vi "p32 zoom algoritmo.vi"() -> ()   [LabVIEW 2013]
panel:
  out "new picture 5":picture
  out "new picture 4":picture
  in  "Numeric 2":dbl
  out "new picture 3":picture
  in  "Numeric":dbl
  out "new picture 2":picture
  in  "path to BMP file":path
  out "new picture":picture
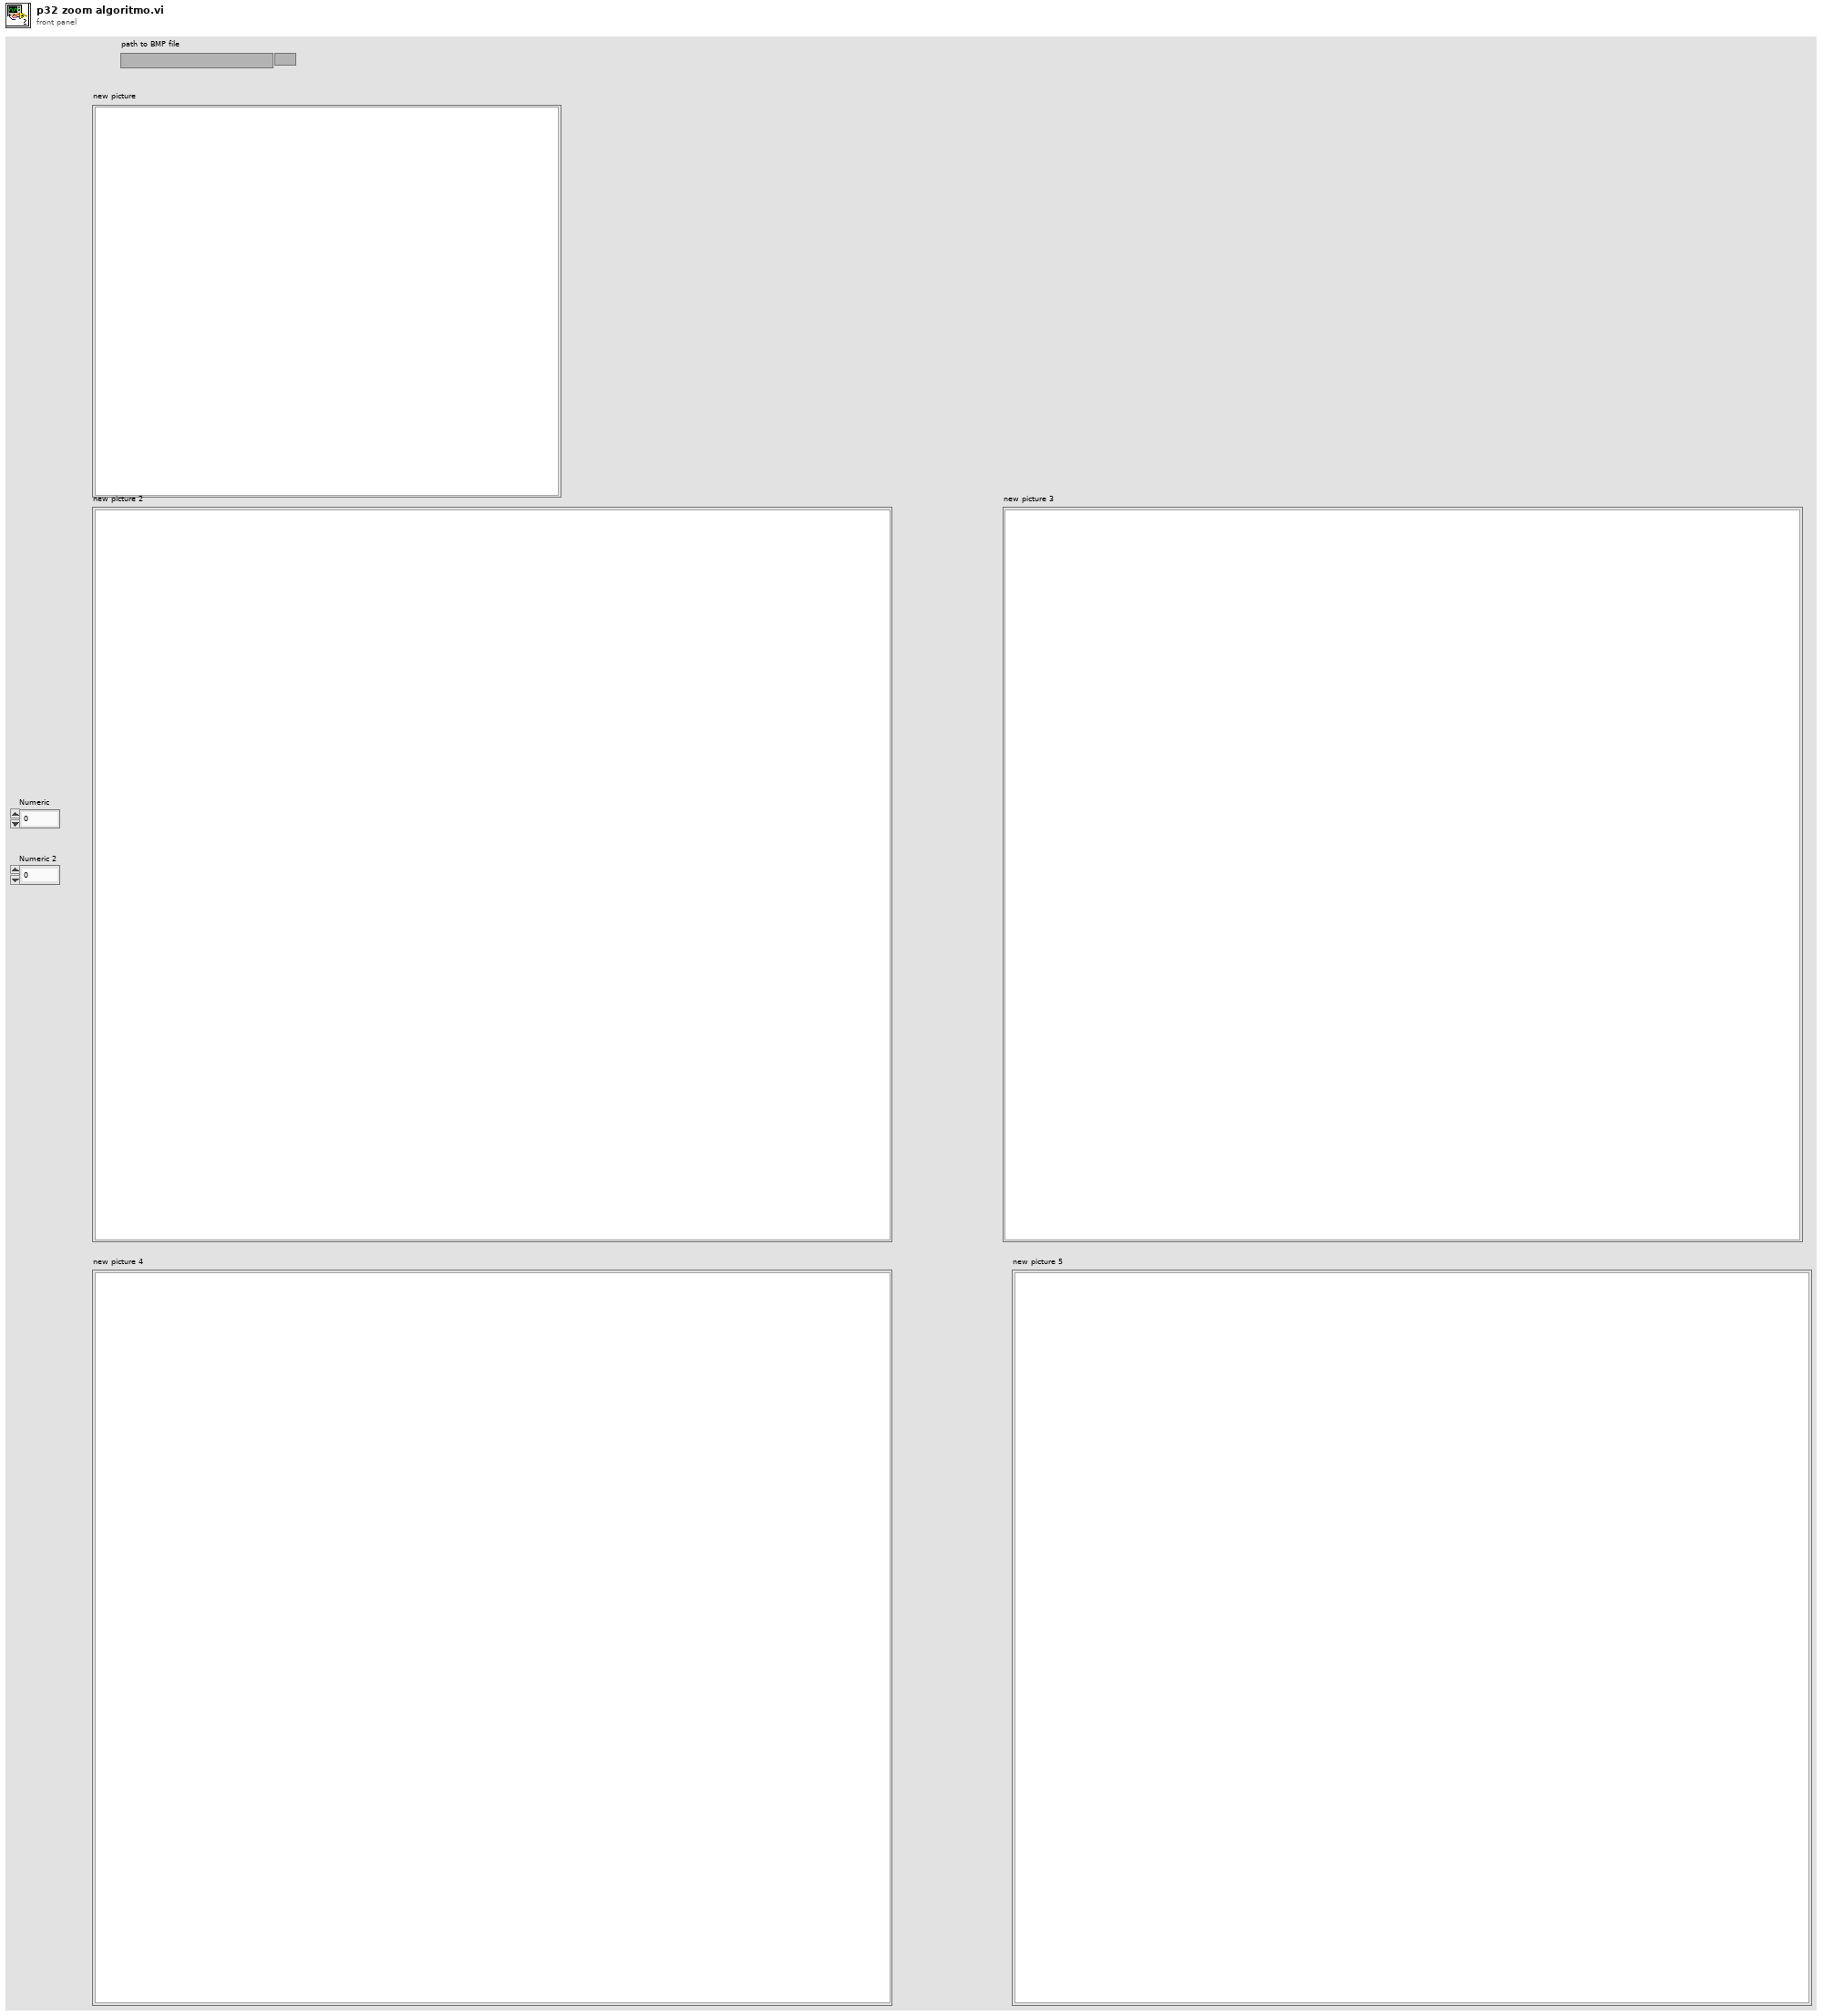
[diagram p1: front panel]
types:
  T1 = typedef "imagedata.ctl" = cluster{"image type":i32, "image depth":i32, "image":u8[], "mask":u8[], "colors":u32[], "Rectangle":cluster{"left":i16, "top":i16, "right":i16, "bottom":i16}}
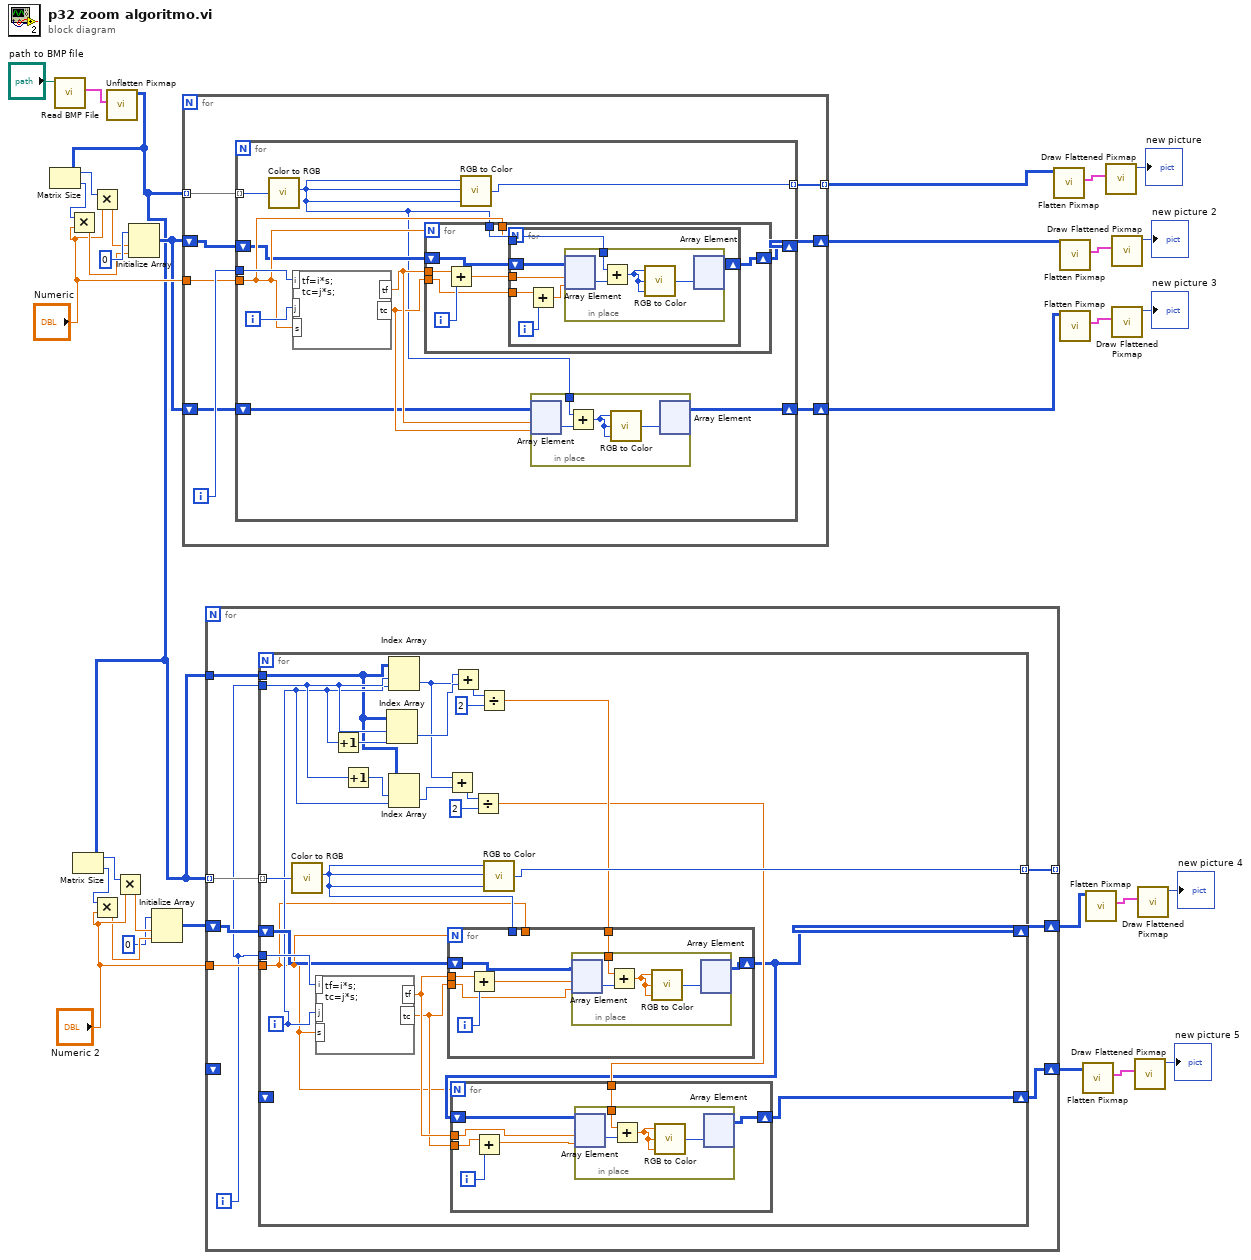
[diagram p0: block diagram]
diagram:
  n1 = call <vilib>:"Read BMP File.vi"("path to BMP file"="path to BMP file") -> ("image data"=w32:T1)  [unwired: 8 in, 2 out]
  n2 = call <vilib>:"Unflatten Pixmap.vi"("image data"=w32) -> ("24-bit pixmap"=w7:u32[][])  [unwired: 4 in, 6 out]
  n3 = Matrix Size(0:w7) -> (1:w23:i32, 2:w22:i32)
  n4 = Multiply(x=w22, y="Numeric") -> (x*y=w20:dbl)
  n5 = Matrix Size(0:w7) -> (1:w9:i32, 2:w10:i32)
  n6 = Multiply(x=w23, y="Numeric") -> (x*y=w21:dbl)
  n7 = Multiply(x=w10, y="Numeric 2") -> (x*y=w12:dbl)
  n8 = Multiply(x=w9, y="Numeric 2") -> (x*y=w11:dbl)
  n9 = Initialize Array(0, w21, w20) -> (w16:i32[][])
  n10 = Initialize Array(0, w11, w12) -> (w14:i32[][])
  n11 = for {
    tunnel: w7 -> [w40] mode=indexing
    tunnel: [w39] -> w30 mode=indexing
    shift-right: [w36] -> w24
    shift-left: w16 -> [w38]
    tunnel: "Numeric" -> [w35]
    shift-right: [w34] -> w15
    shift-left: w16 -> [w33]
    i -> [w37]
    n12 = for {
      tunnel: w40 -> [w52] mode=indexing
      tunnel: [w51] -> w39 mode=indexing
      shift-right: [w50] -> w36
      shift-left: w38 -> [w46]
      tunnel: w37 -> [w49]
      tunnel: w35 -> [w47]
      shift-right: [w42] -> w34
      shift-left: w33 -> [w41]
      i -> [w48]
      n13 = call <vilib>:"Color to RGB.vi"("Color"=w52) -> ("R"=w43:u8)  [unwired: 3 out]
      n14 = formula code="tf=i*s;\ntc=j*s;"("i"=w49, "j"=w48, "s"=w47) -> ("tf"=w45:dbl, "tc"=w44:dbl)
      n15 = for {
        N: w47 -> [_]
        tunnel: w43 -> [w64]
        tunnel: w45 -> [w61]
        tunnel: w44 -> [w58]
        shift-right: [w62] -> w50
        shift-left: w46 -> [w63]
        tunnel: w47 -> [w57]
        i -> [w60]
        n16 = Add(x=w61, y=w60) -> (x+y=w59:dbl)
        n17 = for {
          N: w57 -> [_]
          tunnel: w64 -> [w71]
          tunnel: w59 -> [w68]
          shift-right: [w69] -> w62
          shift-left: w63 -> [w70]
          tunnel: w58 -> [w67]
          i -> [w66]
          n18 = Add(x=w67, y=w66) -> (x+y=w65:dbl)
          n19 = in-place {
            in-place-border: w71 -> [w75]
            n20 = in-place-array #1(w70, w68, w65) -> (w74:i32)
            n21 = Add(x=w75, y=w74) -> (x+y=w72:i32)
            n22 = call <vilib>:"RGB to Color.vi"("B"=w72, "G"=w72, "R"=w72) -> ("Color"=w73:u32)
            n23 = in-place-array #1(w73) -> (w69:i32[][])  [unwired: 2 out]
          }
        }
      }
      n24 = call <vilib>:"RGB to Color.vi"("B"=w43, "G"=w43, "R"=w43) -> ("Color"=w51:u32)
      n25 = in-place {
        in-place-border: w43 -> [w56]
        n26 = in-place-array #2(w41, w45, w44) -> (w55:i32)
        n27 = Add(x=w56, y=w55) -> (x+y=w53:i32)
        n28 = call <vilib>:"RGB to Color.vi"("B"=w53, "G"=w53, "R"=w53) -> ("Color"=w54:u32)
        n29 = in-place-array #2(w54) -> (w42:i32[][])  [unwired: 2 out]
      }
    }
  }
  n30 = for {
    tunnel: w7 -> [w83] mode=indexing
    tunnel: [w82] -> _ mode=indexing
    shift-right: [w80] -> w4
    shift-left: w14 -> [w81]
    tunnel: "Numeric 2" -> [w79]
    tunnel: w7 -> [w78]
    shift-right: [w76] -> w1
    shift-left: _ -> [_]
    i -> [w77]
    n31 = for {
      tunnel: w83 -> [w107] mode=indexing
      tunnel: [w106] -> w82 mode=indexing
      shift-right: [w87] -> w80
      shift-left: w81 -> [w104]
      tunnel: w77 -> [w105]
      tunnel: w79 -> [w84]
      tunnel: w78 -> [w90]
      tunnel: w77 -> [w96]
      shift-right: [w86] -> w76
      shift-left: _ -> [_]
      i -> [w95]
      n32 = call <vilib>:"Color to RGB.vi"("Color"=w107) -> ("R"=w103:u8)  [unwired: 3 out]
      n33 = formula code="tf=i*s;\ntc=j*s;"("i"=w105, "j"=w95, "s"=w84) -> ("tf"=w88:dbl, "tc"=w85:dbl)
      n34 = Increment(x=w95) -> (x+1=w102:i32)
      n35 = Increment(x=w96) -> (x+1=w97:i32)
      n36 = Index Array(array=w90, index (row)=w96, index (col)=w102) -> (element=w101:u32)
      n37 = Index Array(array=w90, index (row)=w96, index (col)=w95) -> (element=w92:u32)
      n38 = Index Array(array=w90, index (row)=w97, index (col)=w95) -> (element=w91:u32)
      n39 = Add(x=w92, y=w91) -> (x+y=w93:u32)
      n40 = Add(x=w92, y=w101) -> (x+y=w100:u32)
      n41 = Divide(x=w93, y=u32 2) -> (x/y=w89:dbl)
      n42 = Divide(x=w100, y=u32 2) -> (x/y=w98:dbl)
      n43 = for {
        N: w84 -> [_]
        tunnel: w103 -> [_]
        tunnel: w88 -> [w125]
        tunnel: w85 -> [w123]
        shift-right: [w119] -> w87
        shift-left: w104 -> [w121]
        tunnel: w84 -> [_]
        tunnel: w98 -> [w120]
        i -> [w124]
        n44 = Add(x=w125, y=w124) -> (x+y=w122:dbl)
        n45 = in-place {
          in-place-border: w120 -> [w126]
          n46 = in-place-array #3(w121, w122, w123) -> (w129:i32)
          n47 = Add(x=w126, y=w129) -> (x+y=w127:dbl)
          n48 = call <vilib>:"RGB to Color.vi"("B"=w127, "G"=w127, "R"=w127) -> ("Color"=w128:u32)
          n49 = in-place-array #3(w128) -> (w119:i32[][])  [unwired: 2 out]
        }
      }
      n50 = for {
        N: w84 -> [_]
        shift-right: [w113] -> w86
        shift-left: w87 -> [w110]
        tunnel: w89 -> [w112]
        tunnel: w88 -> [w108]
        tunnel: w85 -> [w109]
        i -> [w114]
        n51 = Add(x=w109, y=w114) -> (x+y=w111:dbl)
        n52 = in-place {
          in-place-border: w112 -> [w117]
          n53 = in-place-array #4(w110, w108, w111) -> (w116:i32)
          n54 = Add(x=w117, y=w116) -> (x+y=w118:dbl)
          n55 = call <vilib>:"RGB to Color.vi"("B"=w118, "G"=w118, "R"=w118) -> ("Color"=w115:u32)
          n56 = in-place-array #4(w115) -> (w113:i32[][])  [unwired: 2 out]
        }
      }
      n57 = call <vilib>:"RGB to Color.vi"("B"=w103, "G"=w103, "R"=w103) -> ("Color"=w106:u32)
    }
  }
  n58 = call <vilib>:"Flatten Pixmap.vi"("24-bit pixmap"=w30) -> ("image data"=w31:T1)  [unwired: 10 in]
  n59 = call <vilib>:"Flatten Pixmap.vi"("24-bit pixmap"=w24) -> ("image data"=w25:T1)  [unwired: 10 in]
  n60 = call <vilib>:"Flatten Pixmap.vi"("24-bit pixmap"=w15) -> ("image data"=w18:T1)  [unwired: 10 in]
  n61 = call <vilib>:"Flatten Pixmap.vi"("24-bit pixmap"=w1) -> ("image data"=w3:T1)  [unwired: 10 in]
  n62 = call <vilib>:"Flatten Pixmap.vi"("24-bit pixmap"=w4) -> ("image data"=w5:T1)  [unwired: 10 in]
  n63 = call <vilib>:"Draw Flattened Pixmap.vi"("image data"=w31) -> ("new picture"=→"new picture":picture)  [unwired: 8 in]
  n64 = call <vilib>:"Draw Flattened Pixmap.vi"("image data"=w25) -> ("new picture"=→"new picture 2":picture)  [unwired: 8 in]
  n65 = call <vilib>:"Draw Flattened Pixmap.vi"("image data"=w18) -> ("new picture"=→"new picture 3":picture)  [unwired: 8 in]
  n66 = call <vilib>:"Draw Flattened Pixmap.vi"("image data"=w3) -> ("new picture"=→"new picture 5":picture)  [unwired: 8 in]
  n67 = call <vilib>:"Draw Flattened Pixmap.vi"("image data"=w5) -> ("new picture"=→"new picture 4":picture)  [unwired: 8 in]
